vi "Autonomous Independent.vi"() -> ()   [LabVIEW 2014]
doc: "This VI is called when autonomous begins, and will automatically be terminated when autonomous ends. You can carry out timed or sensor driven robot movement independently without needing to return to the caller."
uses:
  <vilib>/Rock Robotics/WPI/Joystick/WPI_JoystickGetSetRefNum.vi
  <vilib>/Rock Robotics/Network Tables/SD Write Numeric Array.vi
  <vilib>/Rock Robotics/Network Tables/SD Read Number.vi
  <vilib>/Rock Robotics/WPI/RobotDrive/WPI_RobotDriveMecanumDrive_Cartesian.vi
panel:
  out "Current Movement, for debugging":T1 {"Z Joystick Value" scale=-1.0..1.0; "Y Joystick Value" scale=1.0..-1.0; "X Joystick Value" scale=-1.0..1.0}
  in  "Array of robot movements":T2(array[cluster]) {"Z Joystick Value" scale=-1.0..1.0; "Y Joystick Value" scale=1.0..-1.0; "X Joystick Value" scale=-1.0..1.0}
  # "Be sure to right-click and choose Data Operations>>Make Current Value default if you want to save the array values with the VI"
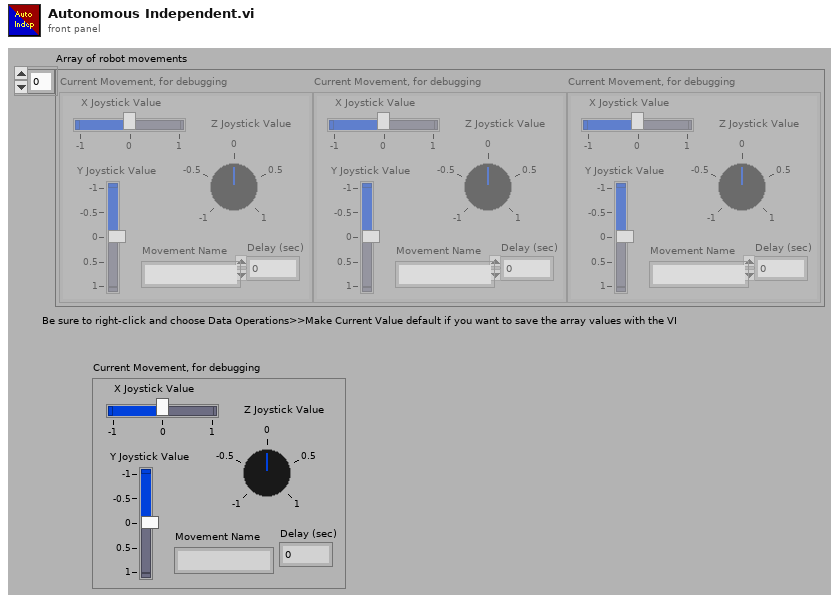
[diagram p1: front panel]
types:
  T1 = cluster{"X Joystick Value":dbl, "Y Joystick Value":dbl, "Z Joystick Value":dbl, "Delay (sec)":dbl, "Movement Name":string}
  T2 = cluster{"X Joystick Value":dbl, "Y Joystick Value":dbl, "Z Joystick Value":dbl, "Delay (sec)":dbl, "Movement Name":string}[]
  T3 = typedef "WPI_RobotDriveDevRef.ctl" = cluster{"DevStatus":errorcluster, "Motors[]":T4[], "Square Inputs":bool, "Max Output":dbl}
  T4 = typedef "WPI_MotorControlDeviceRef.ctl" = cluster{"DeviceStatus":errorcluster, "Type":T5, "PWM":cluster{"Controller":T6, "PWM Channel":T7, "DeadBand":T8}, "CAN":cluster{"Device Number":u8, "Control Mode":T9, "Semaphore":T10, "Max Vout":dbl, "TalonSRX Control Mode":T11}, "Invert":bool, "TransformRef":T12, "InvTransformRef":T12}
  T5 = typedef "WPI_MotorControlType.ctl" = enum16{"PWM", "CAN", "CANTalonSRX"}
  T6 = typedef "FPGA_TypedefDigitalModule.ctl" = enum16{"Controller 1"}
  T7 = typedef "FPGA_DIOPWMChannel.ctl" = enum8{"PWM 0", "PWM 1", "PWM 2", "PWM 3", "PWM 4", "PWM 5", "PWM 6", "PWM 7", "PWM 8", "PWM 9", "PWM MXP 0", "PWM MXP 1", "PWM MXP 2", "PWM MXP 3", "PWM MXP 4", "PWM MXP 5", "PWM MXP 6", "PWM MXP 7", "PWM MXP 8", "PWM MXP 9", "Invalid"}
  T8 = typedef "WPI_PWMDeadband.ctl" = cluster{"Name":string, "maxPositivePwm":i32, "minPositivePwm":i32, "centerPwm":i32, "maxNegativePwm":i32, "minNegativePwm":i32, "angularRange":u16}
  T9 = typedef "WPI_CANJaguar_ControlMode.ctl" = enum8{"Percent VBus", "Current", "Speed", "Position", "Voltage"}
  T10 = typedef "Semaphore RefNum" = refnum<k1>
  T11 = typedef "WPI_CANTalonSRX_APIControlMode.ctl" = enum8{"Percent VBus", "Speed", "Position", "Slave", "Unchanged / Invalid"}
  T12 = typedef "WPI_PWMTransform_ConPane.ctl" = refnum<vi>
  T13 = typedef "WPI_JoystickDevRef.ctl" = cluster{"Device":T14}
  T14 = typedef "WPI_JoystickDeviceEnum.ctl" = enum16{"USB 0", "USB 1", "USB 2", "USB 3", "USB 4", "USB 5"}
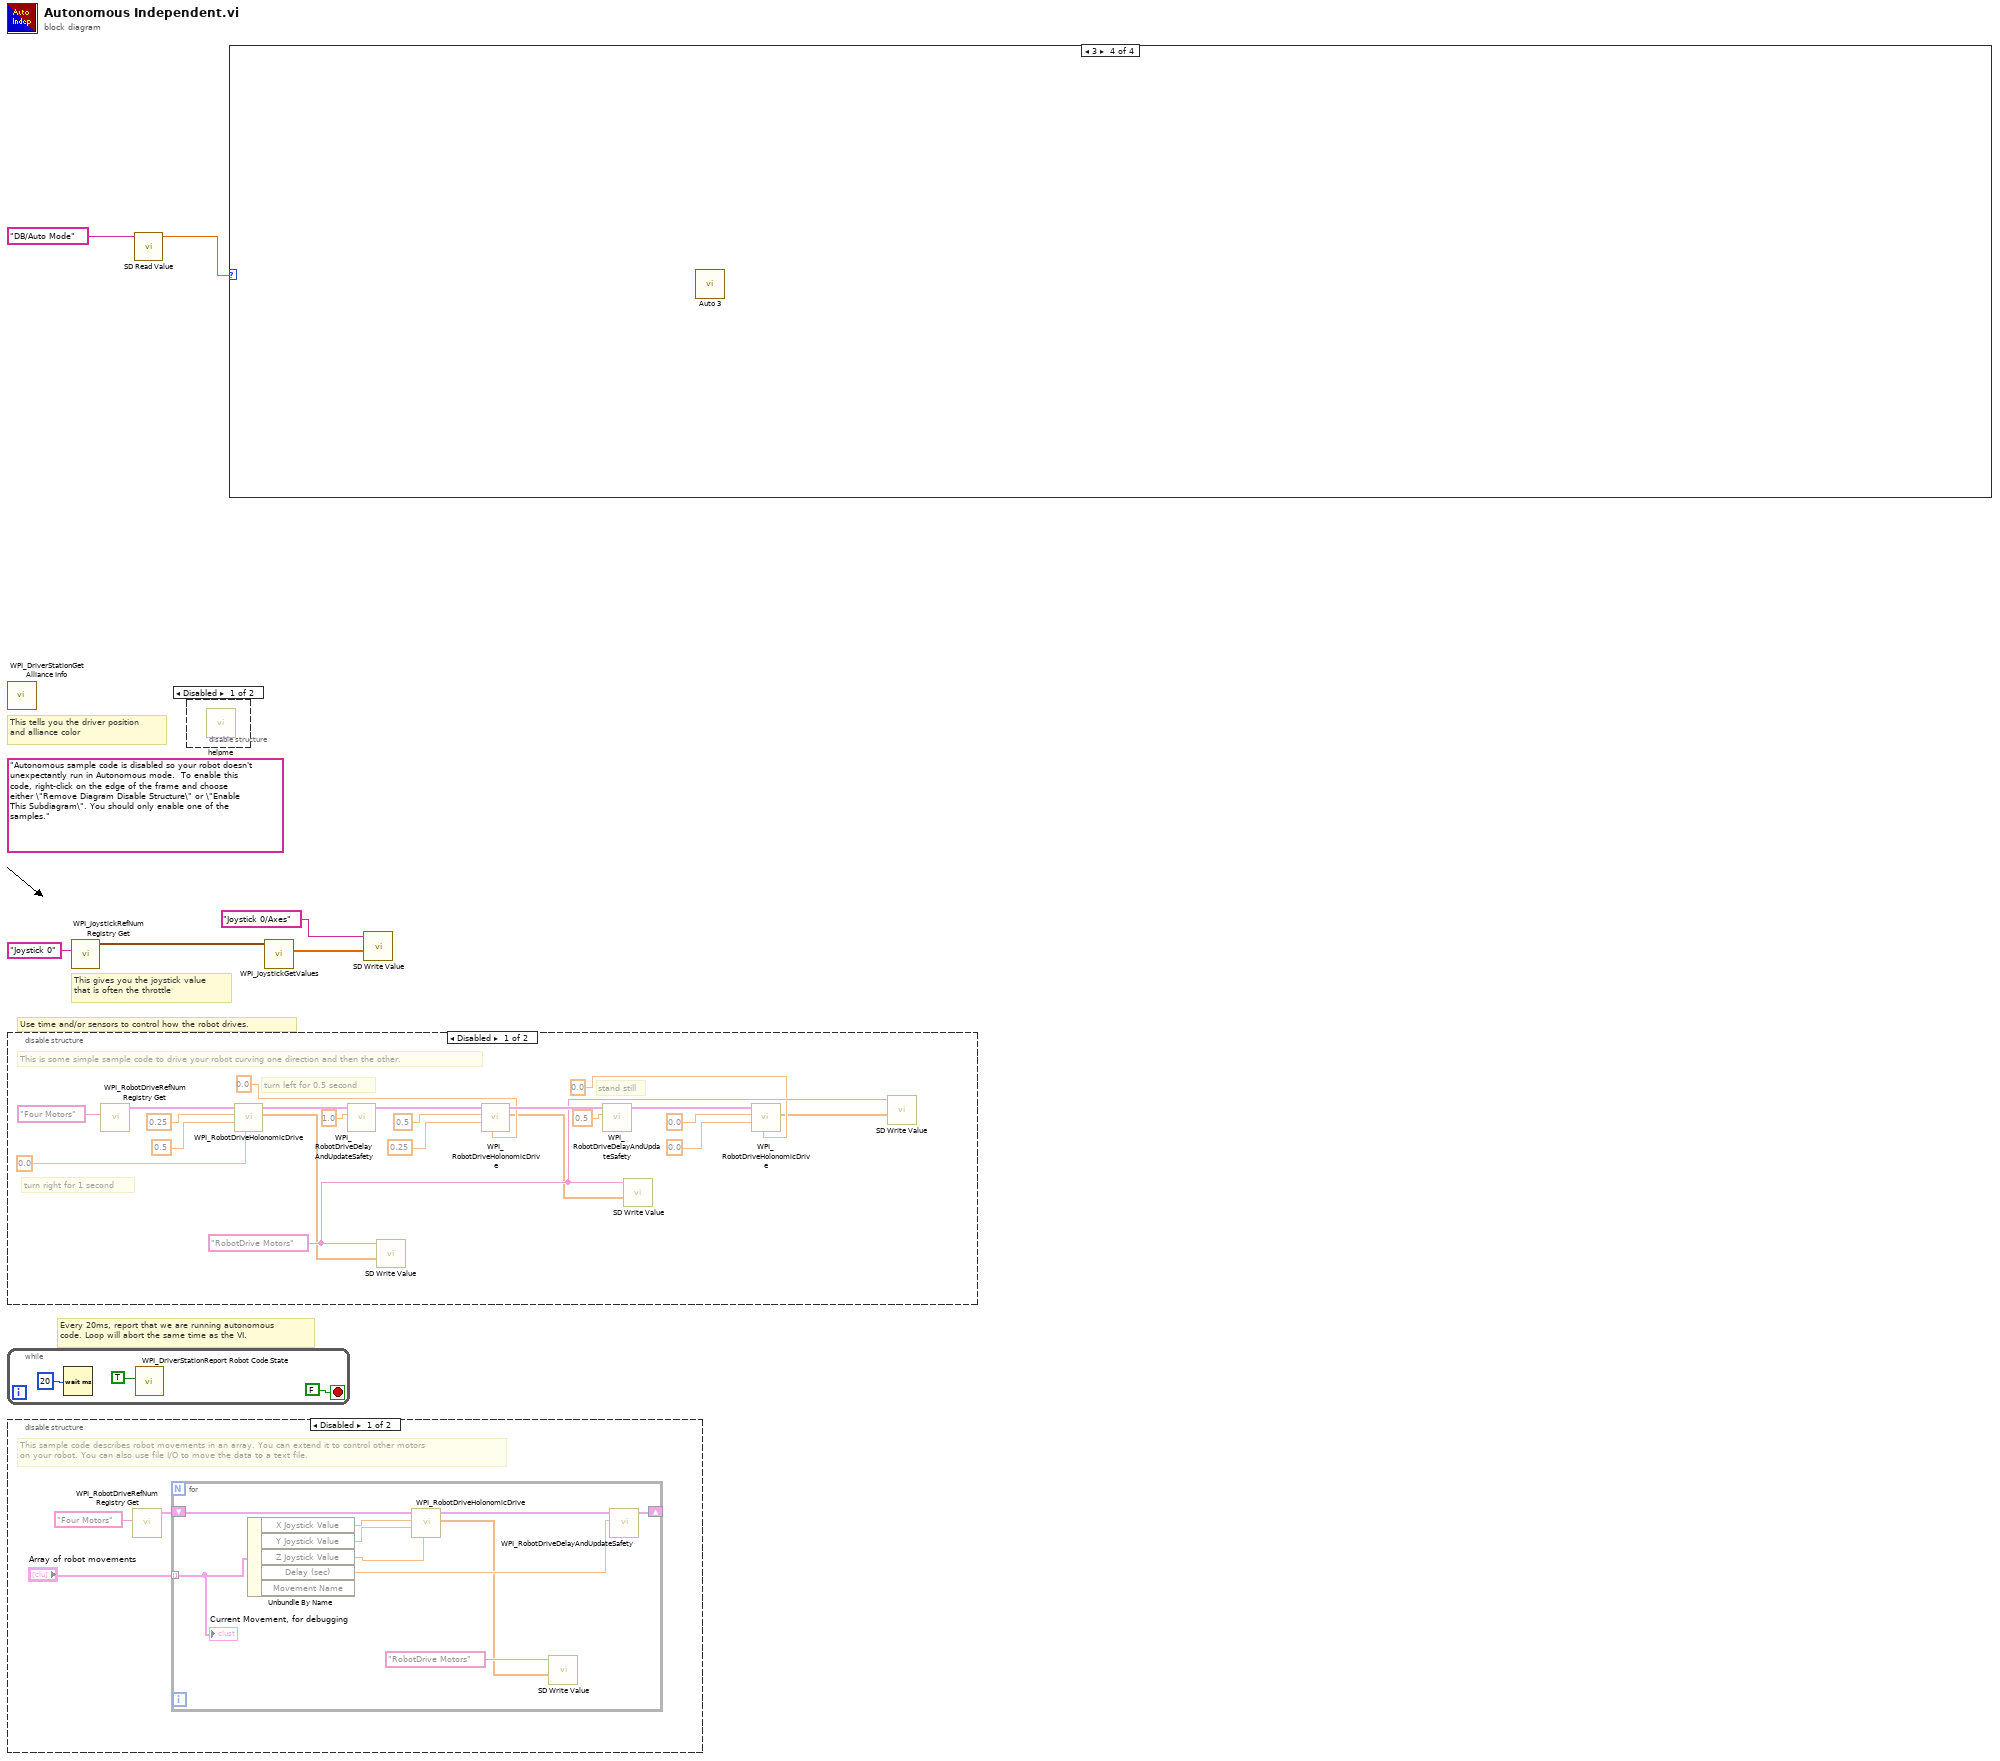
[diagram p0: block diagram]
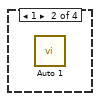
[diagram p3: hidden frame]
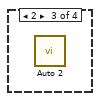
[diagram p4: hidden frame]
diagram:
  (unwired) "Autonomous sample code is disabled so your robot doesn't unexpectantly run in Autonomous mode.  To enable this code, right-click on the edge of the frame and choose either \"Remove Diagram Disable Structure\" or \"Enable This Subdiagram\". You should only enable one of the samples."
  # "Every 20ms, report that we are running autonomous\ncode. Loop will abort the same time as the VI."
  # "This gives you the joystick value\nthat is often the throttle"
  # "Use time and/or sensors to control how the robot drives."
  # "This tells you the driver position\nand alliance color"
  n1 = call <vilib>:"WPI_DriverStationGet Alliance Info.vi"() -> ()  [unwired: 12 out]
  n2 = disable-structure shown="Disabled" {
    frame Disabled {
      w13 = "RobotDrive Motors" ("Name")
      # "This is some simple sample code to drive your robot curving one direction and then the other."
      # "stand still"
      # "turn left for 0.5 second"
      # "turn right for 1 second"
      n3 = call <vilib>:"WPI_RobotDriveRefNum Registry Get.vi"("refnum name"="Four Motors") -> ("RobotDriveDevRef"=w14:T3)  [unwired: 1 in, 9 out]
      n4 = call-poly <vilib>:"WPI_RobotDriveHolonomicDrive.vi"("Rotation"=0.0, "Y"=0.5 ("X axis value"), "X"=0.25 ("X axis value"), "RobotDriveDevRef"=w14) -> ("Motor Values"=w9:dbl[], "RobotDriveDevRef"=w21:T3)  [unwired: 5 in, 1 out]
      n5 = call <vilib>:"WPI_RobotDriveDelayAndUpdateSafety.vi"("Delay (s)"=1.0, "RobotDriveDevRef"=w21) -> ("RobotDriveDevRef 2"=w20:T3)  [unwired: 8 in, 1 out]
      n6 = call-poly <vilib>:"SD Write Value.vi"("Numeric Array"=w9, "Name"=w13) -> ()  [unwired: 8 in, 2 out]
      n7 = call-poly <vilib>:"WPI_RobotDriveHolonomicDrive.vi"("Rotation"=0.0, "Y"=0.25 ("X axis value"), "X"=0.5 ("X axis value"), "RobotDriveDevRef"=w20) -> ("Motor Values"=w8:dbl[], "RobotDriveDevRef"=w19:T3)  [unwired: 5 in, 1 out]
      n8 = call <vilib>:"WPI_RobotDriveDelayAndUpdateSafety.vi"("Delay (s)"=0.5, "RobotDriveDevRef"=w19) -> ("RobotDriveDevRef 2"=w18:T3)  [unwired: 8 in, 1 out]
      n9 = call-poly <vilib>:"SD Write Value.vi"("Numeric Array"=w8, "Name"=w13) -> ()  [unwired: 8 in, 2 out]
      n10 = call-poly <vilib>:"WPI_RobotDriveHolonomicDrive.vi"("Rotation"=0.0 ("X axis value"), "Y"=0.0 ("X axis value"), "X"=0.0 ("X axis value"), "RobotDriveDevRef"=w18) -> ("Motor Values"=w7:dbl[])  [unwired: 5 in, 2 out]
      n11 = call-poly <vilib>:"SD Write Value.vi"("Numeric Array"=w7, "Name"=w13) -> ()  [unwired: 8 in, 2 out]
    }
    frame Enabled {
    }
  }
  n12 = while {
    stop <- FALSE stop-if-true
    n13 = Wait (ms)(milliseconds to wait=u32 20) -> ()  [unwired: 1 out]
    n14 = call <vilib>:"WPI_DriverStationReport Robot Code State.vi"("Autonomous"=TRUE) -> ()  [unwired: 10 in, 1 out]
  }
  n15 = disable-structure shown="Disabled" {
    frame Disabled {
      # "This sample code describes robot movements in an array. You can extend it to control other motors\non your robot. You can also use file I/O to move the data to a text file."
      n16 = call <vilib>:"WPI_RobotDriveRefNum Registry Get.vi"("refnum name"="Four Motors") -> ("RobotDriveDevRef"=w32:T3)  [unwired: 1 in, 9 out]
      n17 = for {
        shift-right: [w40] -> _
        shift-left: w32 -> [w41]
        tunnel: "Array of robot movements" -> [w36] mode=indexing
        n18 = Unbundle By Name(w36) -> ("X Joystick Value"=w39:dbl, "Y Joystick Value"=w38:dbl, "Z Joystick Value"=w35:dbl, "Delay (sec)"=w37:dbl)  [unwired: 1 out]
        n19 = call-poly <vilib>:"WPI_RobotDriveHolonomicDrive.vi"("Rotation"=w35, "Y"=w38, "X"=w39, "RobotDriveDevRef"=w41) -> ("Motor Values"=w34:dbl[], "RobotDriveDevRef"=w42:T3)  [unwired: 5 in, 1 out]
        n20 = call-poly <vilib>:"SD Write Value.vi"("Numeric Array"=w34, "Name"="RobotDrive Motors") -> ()  [unwired: 8 in, 2 out]
        n21 = call <vilib>:"WPI_RobotDriveDelayAndUpdateSafety.vi"("Delay (s)"=w37, "RobotDriveDevRef"=w42) -> ("RobotDriveDevRef 2"=w40:T3)  [unwired: 8 in, 1 out]
        "Current Movement, for debugging" <- w36
      }
    }
    frame Enabled {
    }
  }
  n22 = call <vilib>:"WPI_JoystickRefNum Registry Get.vi"("refnum name"="Joystick 0") -> ("JoystickDevRef"=w5:T13)  [unwired: 1 in, 9 out]
  n23 = call-poly <vilib>:"SD Read Value.vi"("Name"="DB/Auto Mode") -> ("Numeric"=w1:dbl)  [unwired: 8 in, 2 out]
  n24 = disable-structure shown="Disabled" {
    frame Disabled {
      n25 = call "helpme.vi"() -> ()  [unwired: 12 in]
    }
    frame Enabled {
    }
  }
  n26 = case shown="3" w1 {
    frame 0, Default {
    }
    frame 1 {
      n27 = call "Auto 1.vi"() -> ()  [unwired: 11 in, 1 out]
    }
    frame 2 {
      n28 = call "Auto 2.vi"() -> ()  [unwired: 12 in]
    }
    frame 3 {
      n29 = call "Auto 3.vi"() -> ()  [unwired: 11 in, 1 out]
    }
  }
  n30 = call <vilib>:"WPI_JoystickGetValues.vi"("JoystickDevRef"=w5) -> ("Axes"=w3:dbl[])  [unwired: 6 in, 4 out]
  n31 = call-poly <vilib>:"SD Write Value.vi"("Numeric Array"=w3, "Name"="Joystick 0/Axes") -> ()  [unwired: 8 in, 2 out]
